vi "Add Request To Server.vi"(8 "error in":errorcluster, 9 "Room Request":string, 11 "State Cluster":T1) -> (0 "error out":errorcluster)   [LabVIEW 2015]
uses:
  TypeDef/State Cluster.ctl
  LVClasses/Room/Room.lvclass
  LVRestAPI/TypeDef/PostRoomCommands.ctl
  LVClasses/Room/Room.lvclass/Room.ctl
  LVClasses/Room/Read Room Number.vi
  LVRestAPI/RestApi.lvlib
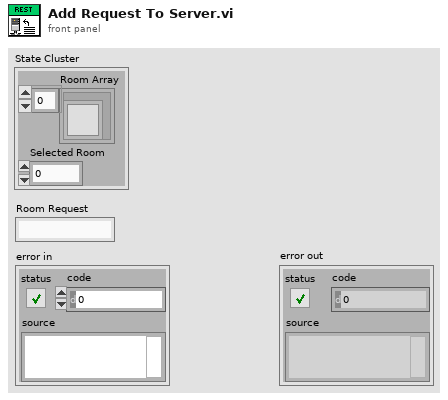
[diagram p1: front panel]
types:
  T1 = typedef "State Cluster.ctl" = cluster{"Room Array":refnum<class "Room.lvclass">[], "Selected Room":u32}
  T2 = typedef "RestApi.lvlib/PostRoomCommands.ctl" = enum16{"WriteFlagState", "WriteFlagColor", "WriteBedVacant", "AddPersonnel", "RemovePersonnel", "AddRequest", "RemoveRequest", "WriteBeaconID", "WriteBedURL"}
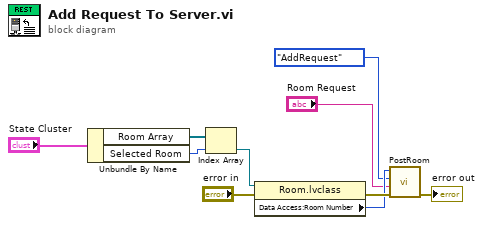
[diagram p0: block diagram]
diagram:
  n1 = Unbundle By Name("State Cluster") -> ("Room Array"=w8:refnum<class "Room.lvclass">[], "Selected Room"=w9:u32)
  n2 = Index Array(array=w8, index=w9) -> (element=w7:refnum<class "Room.lvclass">)
  n3 = property class="Room.lvclass"(reference=w7, error in="error in") -> (error out=w5:errorcluster, "Data Access:Room Number"=w4:i32)  [unwired: 1 out]
  n4 = call "PostRoom.vi"("error in (no error)"=w5, "Data"="Room Request", "Enum"=PostRoomCommands."AddRequest", "Room Number"=w4) -> ("error out"=→"error out":errorcluster)  [unwired: 6 in, 1 out]
